vi "topVI.vi"() -> ()   [LabVIEW 2014]
uses:
  <vilib>/Analysis/NI_AALBase.lvlib
panel:
  out "scored":bool
  out "wrong":i8
  out "correct":i8
  in  "next":bool
  out "phase_saw":dbl
  out "phase_tri":dbl
  out "phase_sin":dbl
  in  "訊號振幅":dbl=0.5
  in  "雜訊振幅":dbl=0.5
  out "原始訊號":string
  in  "stop":bool
  out "max value_saw":dbl
  out "max index_saw":dbl
  out "max value_tri":dbl
  out "max index_tri":dbl
  out "max value_sin":dbl
  out "max index_sin":dbl
  in  "cor_saw":bool
  in  "cor_tri":bool
  in  "cor_sin":bool
  out "鋸齒波":dbl[](graph)
  out "三角波":dbl[](graph)
  out "phase(degree)":dbl
  in  "資料長度":i32=512
  out "signal":dbl[](graph)
  out "弦波":dbl[](graph)
  # "計分"
  # "max index"
  # "max index"
  # "max index"
  # "max value"
  # "max value"
  # "max value"
  # "phase(degree)"
  # "phase(degree)"
  # "phase(degree)"
  # "Ans:"
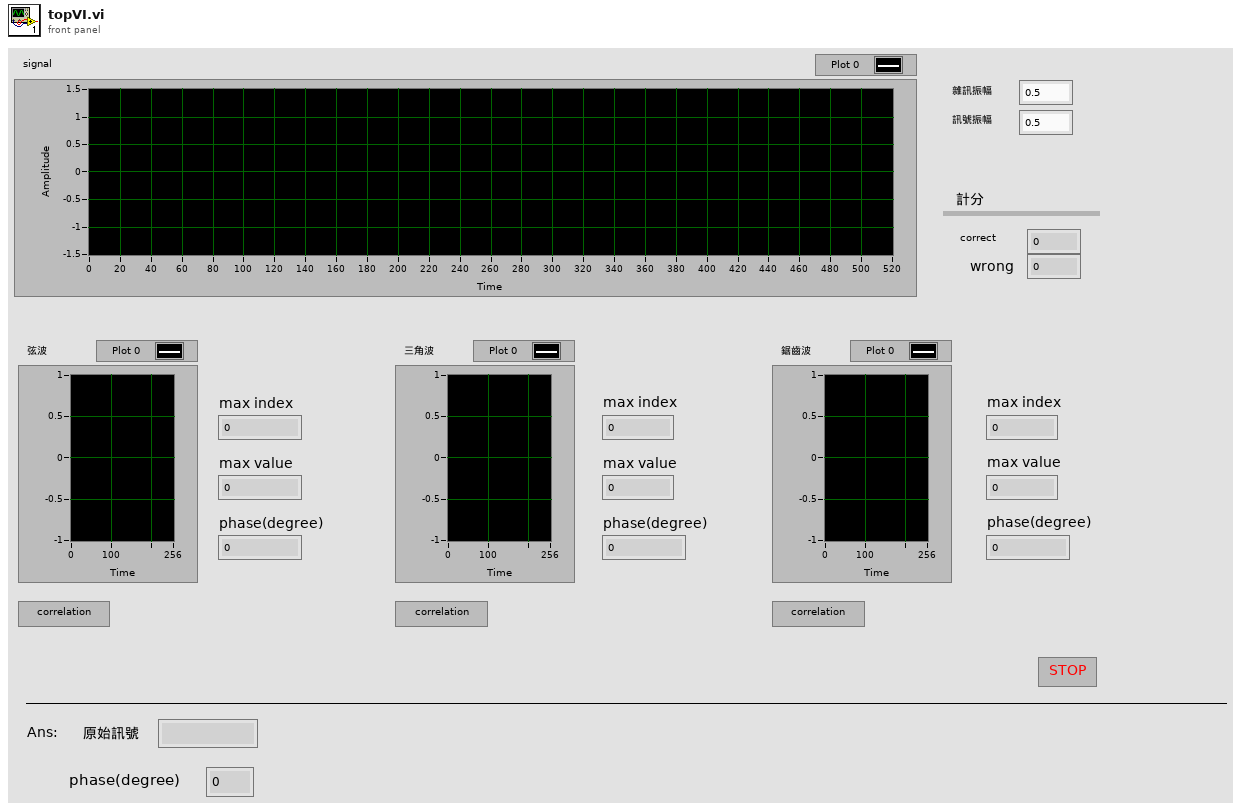
[diagram p1: front panel]
types:
  T1 = enum8{"Enabled", "Disabled", "Disabled and Grayed Out"}
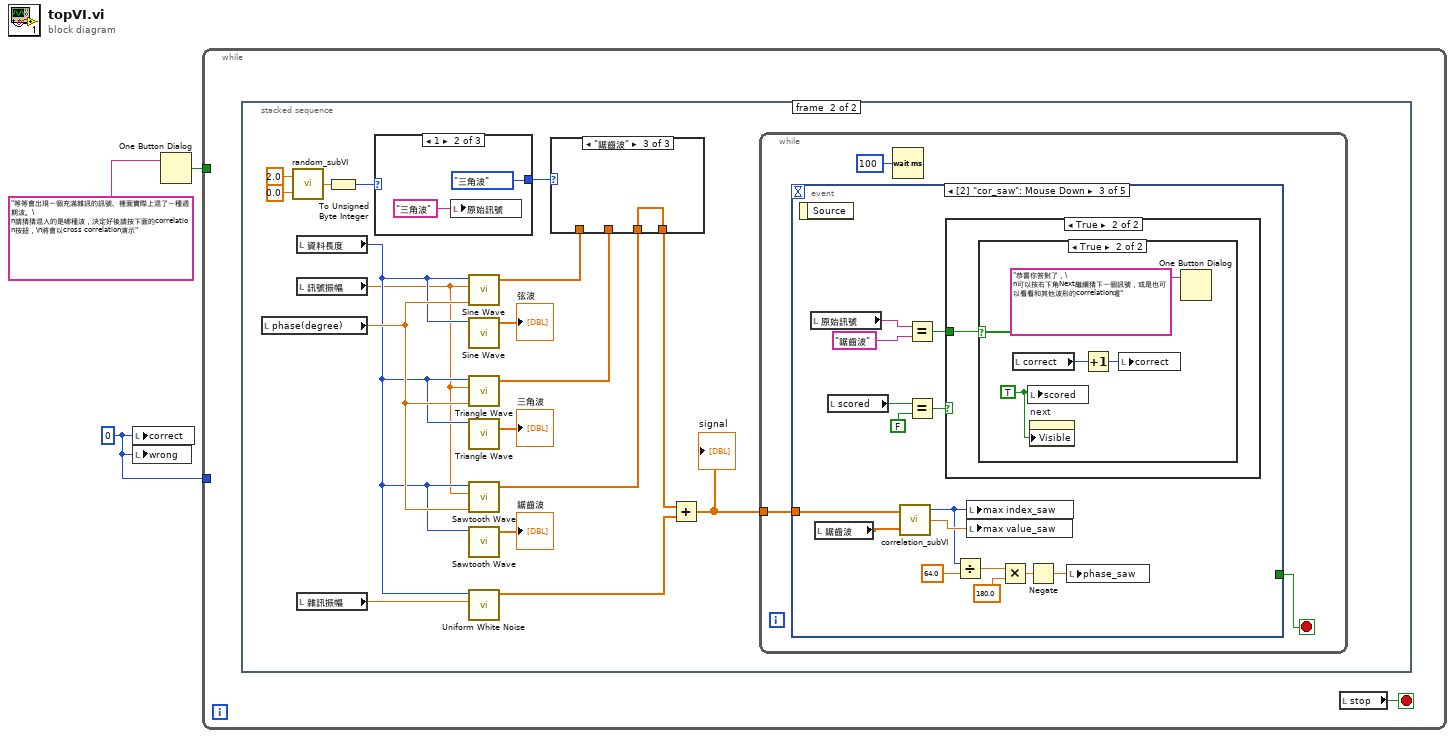
[diagram p0: block diagram]
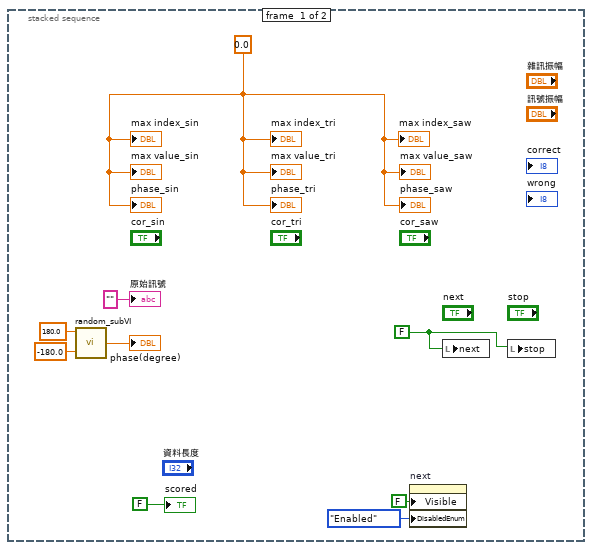
[diagram p2: hidden frame]
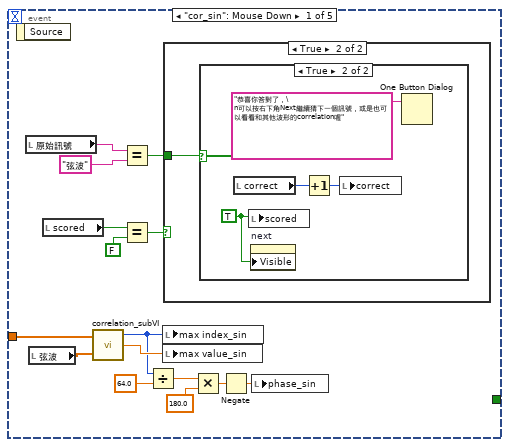
[diagram p3: hidden frame]
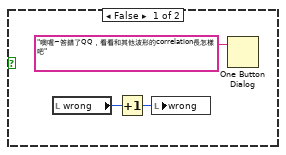
[diagram p5: hidden frame]
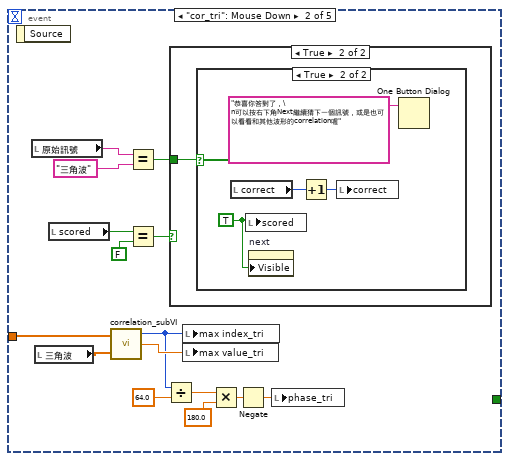
[diagram p6: hidden frame]
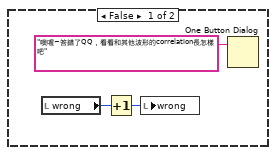
[diagram p8: hidden frame]
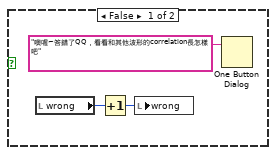
[diagram p10: hidden frame]
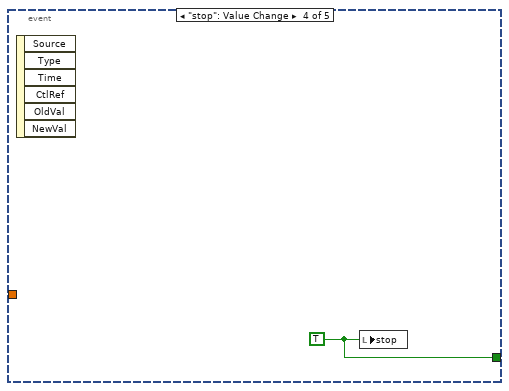
[diagram p11: hidden frame]
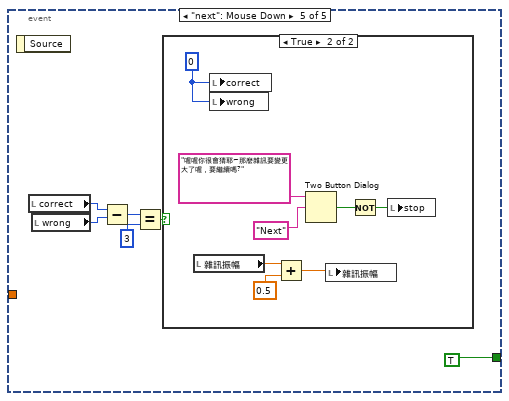
[diagram p12: hidden frame]
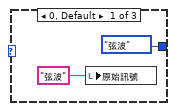
[diagram p14: hidden frame]
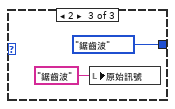
[diagram p15: hidden frame]
diagram:
  w1 = i8 0
  n1 = local write "correct"(w1) -> ()
  n2 = local write "wrong"(w1) -> ()
  n3 = One Button Dialog(message="等等會出現一個充滿雜訊的訊號、裡面實際上混了一種週期波。\n請猜猜混入的是哪種波，決定好後請按下面的correlation按鈕，\n將會以cross correlation演示") -> (true=w2:bool)  [unwired: 1 in]
  n4 = while {
    tunnel: w2 -> [_]
    tunnel: w1 -> [_]
    stop <- w4 stop-if-true
    n5 = stacked-sequence {
      frame #0 {
        w13 = FALSE
        w12 = 0.0
        n6 = call "random_subVI.vi"("lower bound"=-180.0, "upper bound"=180.0) -> ("output"=→"phase(degree)":dbl)
        n7 = property on="next" class="Bool (strict)"("Visible"=FALSE, "DisabledEnum"=T1."Enabled" ("Disabled")) -> ()  [unwired: 2 in, 2 out]
        n8 = local write "next"(w13) -> ()
        n9 = local write "stop"(w13) -> ()
        "max index_saw" <- w12
        "max value_saw" <- w12
        "max index_sin" <- w12
        "max value_sin" <- w12
        "max index_tri" <- w12
        "max value_tri" <- w12
        "原始訊號" <- "" ("String")
        "phase_tri" <- w12
        "phase_saw" <- w12
        "phase_sin" <- w12
        "scored" <- FALSE
      }
      frame #1 {
        n10 = local read "phase(degree)"() -> (w26:dbl)
        n11 = call "random_subVI.vi"("lower bound"=0.0, "upper bound"=2.0) -> ("output"=w29:dbl)
        n12 = local read "資料長度"() -> (w25:i32)
        n13 = local read "訊號振幅"() -> (w16:dbl)
        n14 = local read "雜訊振幅"() -> (w15:dbl)
        n15 = To Unsigned Byte Integer(number=w29) -> (unsigned 8bit integer=w19:u8)
        n16 = case shown="1" w19 {
          tunnel: [enum16{"弦波", "三角波", "鋸齒波"}."弦波" enum16{"弦波", "三角波", "鋸齒波"}."三角波" enum16{"弦波", "三角波", "鋸齒波"}."鋸齒波"] -> w28
          frame 0, Default {
            n17 = local write "原始訊號"("弦波" ("String")) -> ()
          }
          frame 1 {
            n18 = local write "原始訊號"("三角波" ("String")) -> ()
          }
          frame 2 {
            n19 = local write "原始訊號"("鋸齒波" ("String")) -> ()
          }
        }
        n20 = call <vilib>:"Sine Wave.vi"("samples"=w25, "amplitude"=w16, "phase in"=w26) -> ("sine wave"=w18:dbl[])  [unwired: 2 in, 2 out]
        n21 = call <vilib>:"Sine Wave.vi"("samples"=w25) -> ("sine wave"=→"弦波":dbl[])  [unwired: 4 in, 2 out]
        n22 = call <vilib>:"Triangle Wave.vi"("samples"=w25, "amplitude"=w16, "phase in"=w26) -> ("triangle wave"=w21:dbl[])  [unwired: 2 in, 2 out]
        n23 = call <vilib>:"Triangle Wave.vi"("samples"=w25) -> ("triangle wave"=→"三角波":dbl[])  [unwired: 4 in, 2 out]
        n24 = call <vilib>:"Sawtooth Wave.vi"("samples"=w25, "amplitude"=w16, "phase in"=w26) -> ("sawtooth wave"=w24:dbl[])  [unwired: 2 in, 2 out]
        n25 = call <vilib>:"Sawtooth Wave.vi"("samples"=w25) -> ("sawtooth wave"=→"鋸齒波":dbl[])  [unwired: 4 in, 2 out]
        n26 = call <vilib>:"Uniform White Noise.vi"("amplitude"=w15, "samples"=w25) -> ("uniform white noise"=w27:dbl[])  [unwired: 8 in, 1 out]
        n27 = case shown="\"鋸齒波\"" w28 {
          tunnel: w18 -> [w125 _ _]
          tunnel: w24 -> [_ _ w127]
          tunnel: w21 -> [_ w126 _]
          tunnel: [w125 w126 w127] -> w17
          frame "弦波" {
          }
          frame "三角波" {
          }
          frame "鋸齒波" {
          }
        }
        n28 = Add(x=w17, y=w27) -> (x+y=w14:dbl[])
        "signal" <- w14
        n29 = while {
          tunnel: w14 -> [w32]
          stop <- w34 stop-if-true
          n30 = event shown="[2] \"cor_saw\": Mouse Down" {
            selector: _ -> [_ _ _ _ _]
            dyn-events: _ -> [_ _ _ _ _]
            timeout: _ -> [_ _ _ _ _]
            tunnel: [_ _ _ w104 TRUE] -> w34
            tunnel: w32 -> [w43 w66 w89 _ _]
            event "cor_sin": Mouse Down {
              n31 = event-data() -> ()  [unwired: 1 in, 1 out]
              n32 = local read "原始訊號"() -> (w38:string)
              n33 = local read "弦波"() -> (w49:dbl[])
              n34 = local read "scored"() -> (w41:bool)
              n35 = call "correlation_subVI.vi"("signal"=w43, "compare"=w49) -> ("max index"=w44:i32, "max value"=w48:dbl)  [unwired: 1 in, 1 out]
              n36 = Equal?(x=w38, y="弦波") -> (x = y?=w37:bool)
              n37 = Equal?(x=w41, y=FALSE) -> (x = y?=w42:bool)
              n38 = Divide(x=w44, y=64.0) -> (x/y=w47:dbl)
              n39 = local write "max index_sin"(w44) -> ()
              n40 = local write "max value_sin"(w48) -> ()
              n41 = case shown="True" w42 {
                tunnel: w37 -> [_ w50]
                frame False {
                }
                frame True {
                  n42 = case shown="True" w50 {
                    frame False {
                      n43 = local read "wrong"() -> (w53:i8)
                      n44 = Increment(x=w53) -> (x+1=w52:i8)
                      n45 = local write "wrong"(w52) -> ()
                      n46 = One Button Dialog(message="噢喔~答錯了QQ，看看和其他波形的correlation長怎樣吧") -> ()  [unwired: 1 in, 1 out]
                    }
                    frame True {
                      w54 = TRUE
                      n47 = local read "correct"() -> (w57:i8)
                      n48 = local write "scored"(w54) -> ()
                      n49 = property on="next" class="Bool (strict)"("Visible"=w54) -> ()  [unwired: 2 in, 2 out]
                      n50 = Increment(x=w57) -> (x+1=w56:i8)
                      n51 = local write "correct"(w56) -> ()
                      n52 = One Button Dialog(message="恭喜你答對了，\n可以按右下角Next繼續猜下一個訊號，或是也可以看看和其他波形的correlation喔") -> ()  [unwired: 1 in, 1 out]
                    }
                  }
                }
              }
              n53 = Multiply(x=w47, y=180.0) -> (x*y=w36:dbl)
              n54 = Negate(x=w36) -> (-x=w35:dbl)
              n55 = local write "phase_sin"(w35) -> ()
            }
            event "cor_tri": Mouse Down {
              n56 = event-data() -> ()  [unwired: 1 in, 1 out]
              n57 = local read "原始訊號"() -> (w61:string)
              n58 = local read "三角波"() -> (w72:dbl[])
              n59 = local read "scored"() -> (w64:bool)
              n60 = call "correlation_subVI.vi"("signal"=w66, "compare"=w72) -> ("max index"=w67:i32, "max value"=w71:dbl)  [unwired: 1 in, 1 out]
              n61 = Equal?(x=w61, y="三角波") -> (x = y?=w60:bool)
              n62 = Equal?(x=w64, y=FALSE) -> (x = y?=w65:bool)
              n63 = Divide(x=w67, y=64.0) -> (x/y=w70:dbl)
              n64 = case shown="True" w65 {
                tunnel: w60 -> [_ w73]
                frame False {
                }
                frame True {
                  n65 = case shown="True" w73 {
                    frame False {
                      n66 = local read "wrong"() -> (w76:i8)
                      n67 = Increment(x=w76) -> (x+1=w75:i8)
                      n68 = local write "wrong"(w75) -> ()
                      n69 = One Button Dialog(message="噢喔~答錯了QQ，看看和其他波形的correlation長怎樣吧") -> ()  [unwired: 1 in, 1 out]
                    }
                    frame True {
                      w77 = TRUE
                      n70 = local read "correct"() -> (w80:i8)
                      n71 = local write "scored"(w77) -> ()
                      n72 = property on="next" class="Bool (strict)"("Visible"=w77) -> ()  [unwired: 2 in, 2 out]
                      n73 = Increment(x=w80) -> (x+1=w79:i8)
                      n74 = local write "correct"(w79) -> ()
                      n75 = One Button Dialog(message="恭喜你答對了，\n可以按右下角Next繼續猜下一個訊號，或是也可以看看和其他波形的correlation喔") -> ()  [unwired: 1 in, 1 out]
                    }
                  }
                }
              }
              n76 = local write "max index_tri"(w67) -> ()
              n77 = local write "max value_tri"(w71) -> ()
              n78 = Multiply(x=w70, y=180.0) -> (x*y=w59:dbl)
              n79 = Negate(x=w59) -> (-x=w58:dbl)
              n80 = local write "phase_tri"(w58) -> ()
            }
            event "cor_saw": Mouse Down {
              n81 = event-data() -> ()  [unwired: 1 in, 1 out]
              n82 = local read "原始訊號"() -> (w87:string)
              n83 = local read "鋸齒波"() -> (w95:dbl[])
              n84 = local read "scored"() -> (w84:bool)
              n85 = call "correlation_subVI.vi"("signal"=w89, "compare"=w95) -> ("max index"=w90:i32, "max value"=w94:dbl)  [unwired: 1 in, 1 out]
              n86 = Equal?(x=w87, y="鋸齒波") -> (x = y?=w88:bool)
              n87 = Equal?(x=w84, y=FALSE) -> (x = y?=w83:bool)
              n88 = case shown="True" w83 {
                tunnel: w88 -> [_ w96]
                frame False {
                }
                frame True {
                  n89 = case shown="True" w96 {
                    frame False {
                      n90 = local read "wrong"() -> (w99:i8)
                      n91 = Increment(x=w99) -> (x+1=w98:i8)
                      n92 = local write "wrong"(w98) -> ()
                      n93 = One Button Dialog(message="噢喔~答錯了QQ，看看和其他波形的correlation長怎樣吧") -> ()  [unwired: 1 in, 1 out]
                    }
                    frame True {
                      w100 = TRUE
                      n94 = local read "correct"() -> (w103:i8)
                      n95 = local write "scored"(w100) -> ()
                      n96 = property on="next" class="Bool (strict)"("Visible"=w100) -> ()  [unwired: 2 in, 2 out]
                      n97 = Increment(x=w103) -> (x+1=w102:i8)
                      n98 = local write "correct"(w102) -> ()
                      n99 = One Button Dialog(message="恭喜你答對了，\n可以按右下角Next繼續猜下一個訊號，或是也可以看看和其他波形的correlation喔") -> ()  [unwired: 1 in, 1 out]
                    }
                  }
                }
              }
              n100 = Divide(x=w90, y=64.0) -> (x/y=w93:dbl)
              n101 = local write "max index_saw"(w90) -> ()
              n102 = local write "max value_saw"(w94) -> ()
              n103 = Multiply(x=w93, y=180.0) -> (x*y=w82:dbl)
              n104 = Negate(x=w82) -> (-x=w81:dbl)
              n105 = local write "phase_saw"(w81) -> ()
            }
            event "stop": Value Change {
              w104 = TRUE
              n106 = event-data() -> ()  [unwired: 1 in, 6 out]
              n107 = local write "stop"(w104) -> ()
            }
            event "next": Mouse Down {
              n108 = event-data() -> ()  [unwired: 1 in, 1 out]
              n109 = local read "correct"() -> (w109:i8)
              n110 = local read "wrong"() -> (w108:i8)
              n111 = Subtract(x=w109, y=w108) -> (x-y=w107:i8)
              n112 = Equal?(x=w107, y=i8 3) -> (x = y?=w105:bool)
              n113 = case shown="True" w105 {
                frame False {
                }
                frame True {
                  w118 = i8 0
                  n114 = local read "雜訊振幅"() -> (w117:dbl)
                  n115 = local write "correct"(w118) -> ()
                  n116 = local write "wrong"(w118) -> ()
                  n117 = Add(x=w117, y=0.5) -> (x+y=w115:dbl)
                  n118 = Two Button Dialog(message="喔喔你很會猜耶~那麼雜訊要變更大了喔，要繼續嗎?", 2:"Next" ("T button name (\"OK\")")) -> (T button?=w112:bool)  [unwired: 1 in]
                  n119 = local write "雜訊振幅"(w115) -> ()
                  n120 = Not(x=w112) -> (.not. x?=w111:bool)
                  n121 = local write "stop"(w111) -> ()
                }
              }
            }
          }
          n122 = Wait (ms)(milliseconds to wait=u32 100) -> ()  [unwired: 1 out]
        }
      }
    }
    n123 = local read "stop"() -> (w4:bool)
  }
